vi "Run Logger Daemon.vi"(8 "Error In":errorcluster, 11 "TDMS Log In":refnum<class "TDMS Logger.lvclass">) -> (0 "Error Out":errorcluster, 3 "TDMS Log Out":refnum<class "TDMS Logger.lvclass">)   [LabVIEW 2014, in "TDMS Logger.lvlib" / "TDMS Logger.lvclass"]
uses:
  TDMS Logger.lvclass
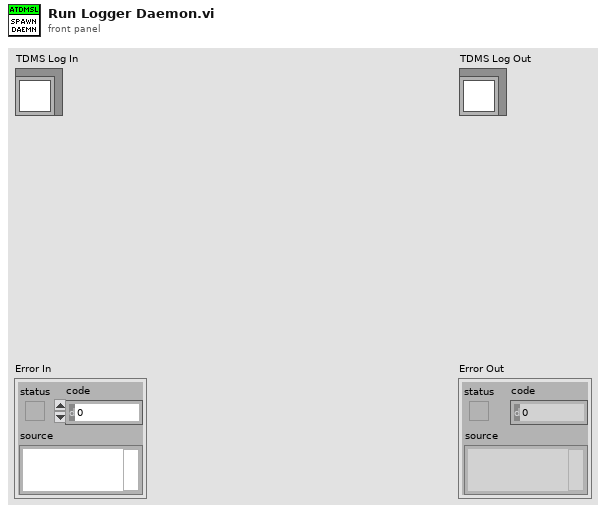
[diagram p1: front panel]
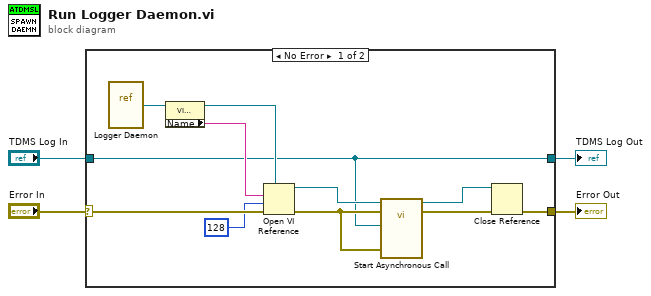
[diagram p0: block diagram]
diagram:
  n1 = case shown="No Error" "Error In" {
    selector: "Error In" -> [w12 w17]
    tunnel: [w5 w17] -> w3
    tunnel: [w8 w16] -> w1
    tunnel: "TDMS Log In" -> [w8 w16]
    frame No Error {
      n2 = vi-ref "Logger Daemon.vi"() -> (w15:refnum<vi>)
      n3 = property class="VI (strict)"(reference=w15) -> (reference out=w14:refnum<vi>, "Name"=w13:string)  [unwired: 1 in, 1 out]
      n4 = Open VI Reference(type specifier VI Refnum (for type only)=w14, vi path=w13, options=128, error in (no error)=w12) -> (vi reference=w10:refnum<vi>, error out=w9:errorcluster)  [unwired: 2 in]
      n5 = call-by-ref "Start Asynchronous Call"(reference=w10, error in=w9, "Error In"=w9, "TDMS Log In"=w8) -> (reference out=w6:refnum<vi>, error out=w7:errorcluster)  [unwired: 10 in]
      n6 = Close Reference(reference=w6, error in (no error)=w7) -> (error out=w5:errorcluster)
    }
    frame Error {
    }
  }
  "Error Out" <- w3
  "TDMS Log Out" <- w1
